vi "record.vi"(0 "Camera in":refnum<class "Camera.lvclass">, 5 "num_images":u32=1, 7 "record_mode":T1(ring), 9 "file_path":path, 11 "error in (no error)":errorcluster) -> (4 "Camera out":refnum<class "Camera.lvclass">, 15 "error out":errorcluster)   [LabVIEW 2020, in "Camera.lvclass"]
doc: "Creates, configures, and starts a new recorder instance. The entire camera configuration must be\nset before calling record.vi. The set_exposure_time.vi is the only exception. This function\nhas no effect on the recorder object and can be called during the recording."
uses:
  Camera.lvclass
  Camera.lvclass/Camera.ctl
  Recorder.lvlib
  GeneralCameraControl.lvlib
  RecordingControl.lvlib
  ImageSensor.lvlib
  Convert.lvlib
panel:
  out "filemode_no_overwrite":bool
  out "blocking_int":bool
  out "recType_int":u16
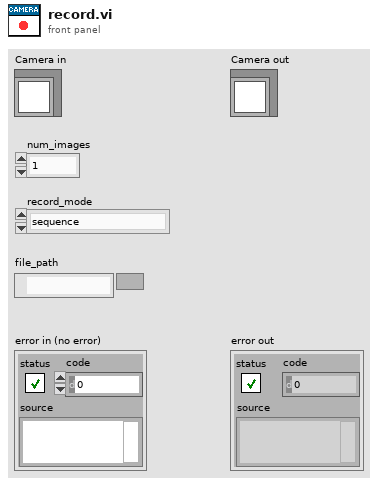
[diagram p1: front panel]
types:
  T1 = enum16{"sequence", "sequence non blocking", "ring buffer", "fifo", "sequence_dpcore", "sequence_non_blocking_dpcore", "ring_buffer_dpcore", "fifo_dpcore", "tif", "multitif", "pcoraw", "b16", "dicom", "multidicom"}
  T2 = map{enum16{"Undefined", "Mono8", "Mono16", "BGRA8", "RGBA8", "BGRA16", "RGBA16", "CompressedMono8"}, bool}
  T3 = cluster{"wSensorTypeDESC":u16, "wSensorSubTypeDESC":u16, "wMaxHorzResStdDESC":u16, "wMaxVertResStdDESC":u16, "wMaxHorzResExtDESC":u16, "wMaxVertResExtDESC":u16, "wDynResDESC":u16, "wMaxBinHorzDESC":u16, "wBinHorzSteppingDESC":u16, "wMaxBinVertDESC":u16, "wBinVertSteppingDESC":u16, "wRoiHorStepsDESC":u16, "wRoiVertStepsDESC":u16, "wNumADCsDESC":u16, "wMinSizeHorzDESC":u16, "dwPixelRateDESC":u32[], "wConvFactDESC":u16[], "sCoolingSetpoints":i16[], "wSoftRoiHorStepsDESC":u16, "wSoftRoiVertStepsDESC":u16, "wIRDESC":u16, "wMinSizeVertDESC":u16, "dwMinDelayDESC":u32, "dwMaxDelayDESC":u32, "dwMinDelayStepDESC":u32, "dwMinExposureDESC":u32, "dwMaxExposureDESC":u32, "dwMinExposureStepDESC":u32, "dwMinDelayIRDESC":u32, "dwMaxDelayIRDESC":u32, "dwMinExposureIRDESC":u32, "dwMaxExposureIRDESC":u32, "wTimeTableDESC":u16, "wDoubleImageDESC":u16, "sMinCoolSetDESC":i16, "sMaxCoolSetDESC":i16, "sDefaultCoolSetDESC":i16, "wPowerDownModeDESC":u16, "wOffsetRegulationDESC":u16, "wColorPatternDESC":u16, "wPatternTypeDESC":u16, "wNumCoolingSetpoints":u16, "dwGeneralCapsDESC1":u32, "dwGeneralCapsDESC2":u32, "dwExtSyncFrequency":u32[], "dwGeneralCapsDESC3":u32, "dwGeneralCapsDESC4":u32}
  T4 = cluster{"iConversionFactor":i32, "iDataBits":i32, "iSensorInfoBits":i32, "iDarkOffset":i32, "strColorCoeff":dbl[], "iCamNum":i32, "hCamera":u64}
  T5 = map{enum16{"Undefined", "Mono8", "Mono16", "BGRA8", "RGBA8", "BGRA16", "RGBA16", "CompressedMono8"}, u64}
  T6 = enum16{"Undefined", "Mono8", "Mono16", "BGRA8", "RGBA8", "BGRA16", "RGBA16", "CompressedMono8"}
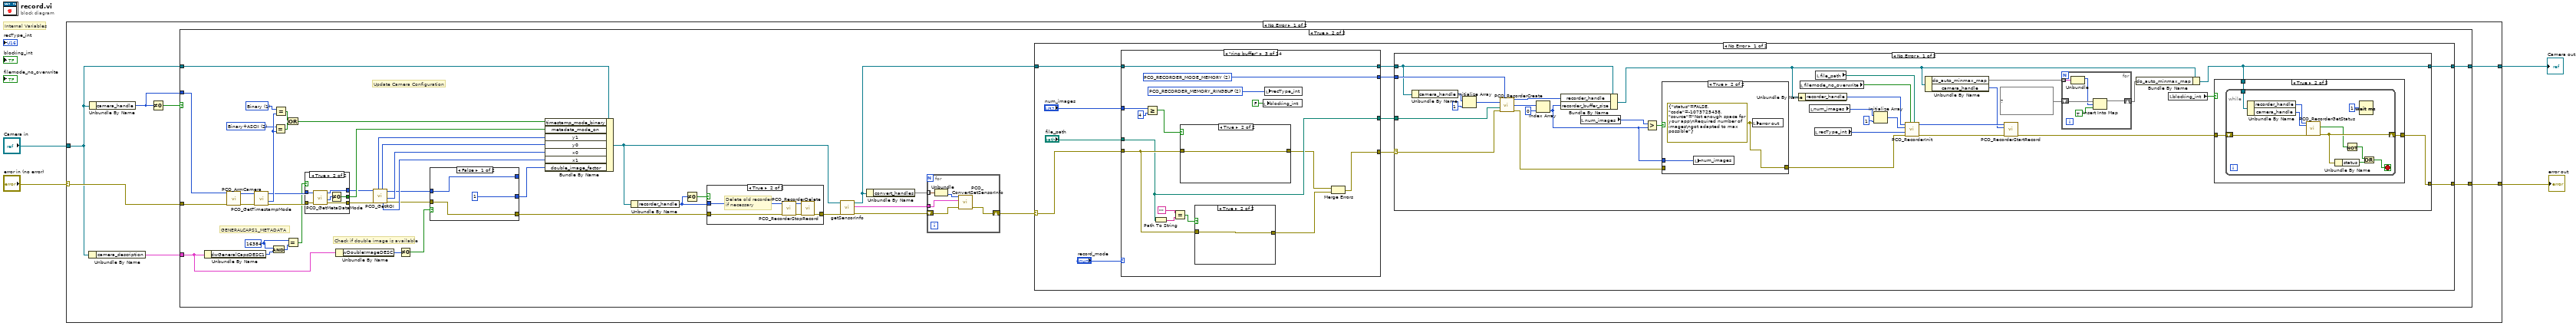
[diagram p0: block diagram]
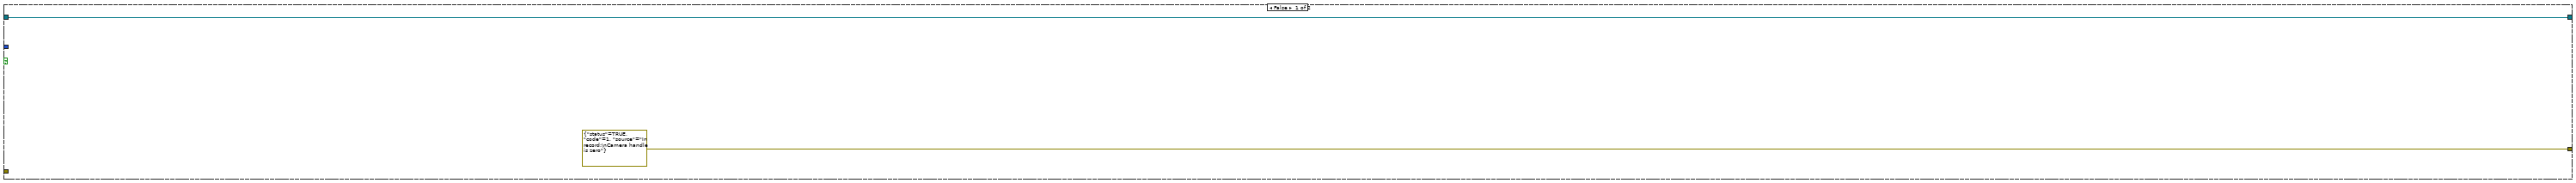
[diagram p2: hidden frame]
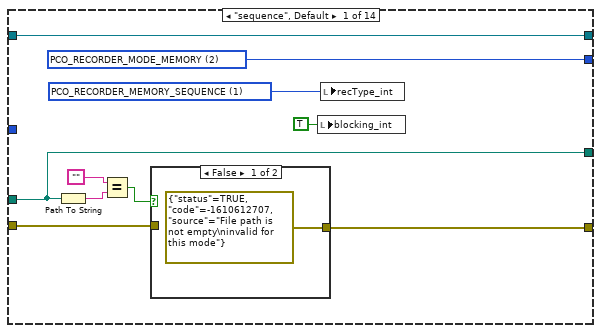
[diagram p6: hidden frame]
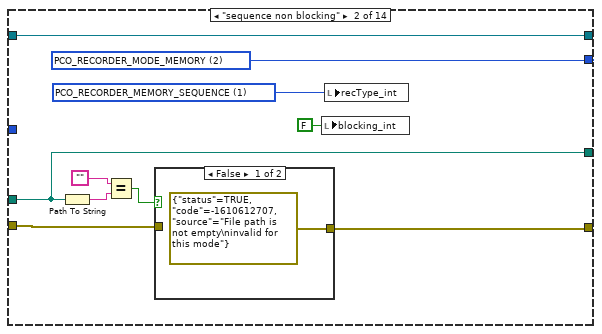
[diagram p8: hidden frame]
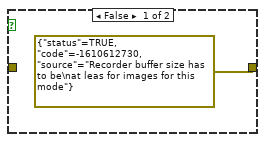
[diagram p10: hidden frame]
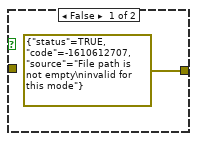
[diagram p11: hidden frame]
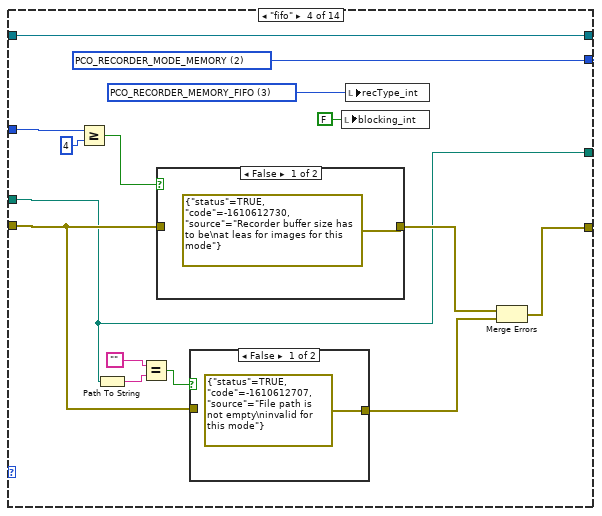
[diagram p12: hidden frame]
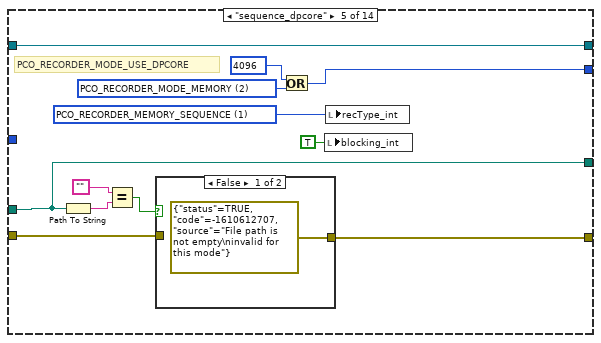
[diagram p15: hidden frame]
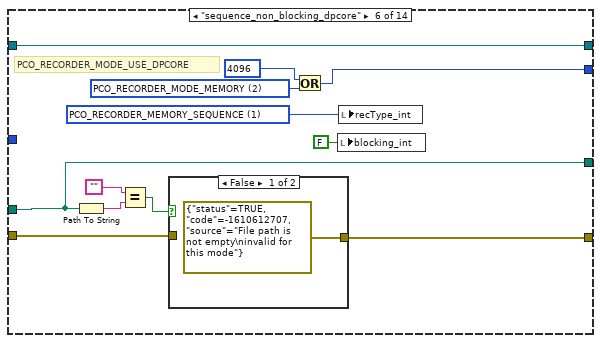
[diagram p17: hidden frame]
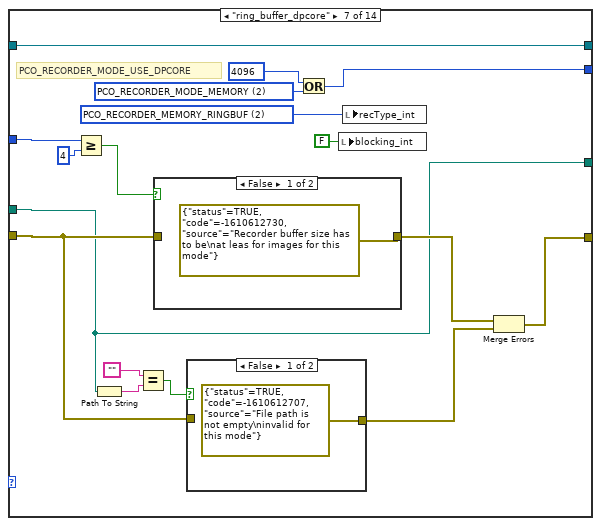
[diagram p19: hidden frame]
diagram:
  # "Internal Variables"
  n1 = case shown="No Error" "error in (no error)" {
    selector: "error in (no error)" -> [w7 w405]
    tunnel: [w10 w405] -> w3
    tunnel: [w9 w404] -> w1
    tunnel: "Camera in" -> [w6 w404]
    frame No Error {
      n2 = Unbundle By Name(w6) -> ("camera_description"=w5:T3)
      n3 = Unbundle By Name(w6) -> ("camera_handle"=w8:u64)
      n4 = Not Equal To 0?(x=w8) -> (x != 0?=w11:bool)
      n5 = case shown="True" w11 {
        tunnel: [errorcluster {"status"=TRUE, "code"=1, "source"="In record:\nCamera handle is zero"} ("error constant") w16] -> w10
        tunnel: w7 -> [_ w54]
        tunnel: w6 -> [w12 w51]
        tunnel: [w12 w14] -> w9
        tunnel: w8 -> [_ w55]
        tunnel: w5 -> [_ w31]
        frame False {
        }
        frame True {
          w40 = u32 16384 ("dwGeneralCapsDESC1")
          w48 = u16 2 items=["OFF", "Binary", "Binary+ASCII", "ASCII"] ("wTimeStampMode")
          w50 = u16 1 items=["OFF", "Binary", "Binary+ASCII", "ASCII"] ("wTimeStampMode")
          # "Update Camera Configuration"
          # "Check if double image is available"
          # "GENERALCAPS1_METADATA"
          n6 = Unbundle By Name(w31) -> ("dwGeneralCapsDESC1"=w42:u32)
          n7 = call "PCO_ArmCamera.vi"("error in (no error)"=w54, "ph"=w55) -> ("error out"=w53:errorcluster, "ph out"=w52:u64)  [unwired: 7 in, 1 out]
          n8 = call "PCO_GetTimestampMode.vi"("error in (no error)"=w53, "ph"=w52) -> ("error out"=w43:errorcluster, "wTimeStampMode"=w49:u16, "ph out"=w44:u64)  [unwired: 6 in, 1 out]
          n9 = And(x=w40, y=w42) -> (x .and. y?=w41:u32)
          n10 = Equal?(x=w48, y=w49) -> (x = y?=w47:bool)
          n11 = Equal?(x=w50, y=w49) -> (x = y?=w46:bool)
          n12 = Or(x=w46, y=w47) -> (x .or. y?=w45:bool)
          n13 = Equal?(x=w40, y=w41) -> (x = y?=w39:bool)
          n14 = case shown="True" w39 {
            tunnel: w44 -> [w395 w403]
            tunnel: w43 -> [w396 w402]
            tunnel: [w395 w401] -> w37
            tunnel: [w396 w400] -> w36
            tunnel: [FALSE w398] -> w38
            frame False {
            }
            frame True {
              n15 = call "PCO_GetMetaDataMode.vi"("error in (no error)"=w402, "ph"=w403) -> ("error out"=w400:errorcluster, "wMetaDataMode"=w399:u16, "ph out"=w401:u64)  [unwired: 4 in, 3 out]
              n16 = Not Equal To 0?(x=w399) -> (x != 0?=w398:bool)
            }
          }
          n17 = Unbundle By Name(w31) -> ("wDoubleImageDESC"=w30:u16)
          n18 = call "PCO_GetROI.vi"("error in (no error)"=w36, "ph"=w37) -> ("error out"=w28:errorcluster, "wRoiX0"=w33:u16, "ph out"=w27:u64, "wRoiX1"=w32:u16, "wRoiY0"=w35:u16, "wRoiY1"=w34:u16)  [unwired: 3 in, 1 out]
          n19 = Not Equal To 0?(x=w30) -> (x != 0?=w29:bool)
          n20 = case shown="False" w29 {
            tunnel: w28 -> [w383 w392]
            tunnel: w27 -> [w384 w391]
            tunnel: [u16 1 ("double_image_factor") w388] -> w26
            tunnel: [w383 w387] -> w25
            tunnel: [w384 w386] -> _
            frame False {
            }
            frame True {
              n21 = call "PCO_GetDoubleImageMode.vi"("error in (no error)"=w392, "ph"=w391) -> ("error out"=w387:errorcluster, "wDoubleImage"=w390:u16, "ph out"=w386:u64)  [unwired: 6 in, 1 out]
              n22 = Not Equal To 0?(x=w390) -> (x != 0?=w389:bool)
              n23 = case shown="True" w389 {
                tunnel: [u16 1 ("double_image_factor") u16 2 ("double_image_factor")] -> w388
                frame False {
                }
                frame True {
                }
              }
            }
          }
          n24 = Bundle By Name(cluster=w51, "timestamp_mode_binary"=w45, "metadata_mode_on"=w38, "y1"=w34, "y0"=w35, "x0"=w33, "x1"=w32, "double_image_factor"=w26) -> (w21:refnum<class "Camera.lvclass">)
          n25 = Unbundle By Name(w21) -> ("recorder_handle"=w23:u64)
          n26 = Not Equal To 0?(x=w23) -> (x != 0?=w24:bool)
          n27 = case shown="True" w24 {
            tunnel: w23 -> [_ w381]
            tunnel: w25 -> [w377 w382]
            tunnel: [w377 w378] -> w22
            frame False {
            }
            frame True {
              # "Delete old recorder\nif necessary"
              n28 = call "PCO_RecorderStopRecord.vi"("error in (no error)"=w382, "phRec"=w381) -> ("error out"=w380:errorcluster, "phRec out"=w379:u64)  [unwired: 7 in, 1 out]
              n29 = call "PCO_RecorderDelete.vi"("error in (no error)"=w380, "phRec"=w379) -> ("error out"=w378:errorcluster)  [unwired: 8 in, 1 out]
            }
          }
          n30 = call-dynamic "getSensorInfo.vi"("error in (no error)"=w22, "Camera in"=w21) -> ("error out"=w18:errorcluster, "PCO_SensorInfo"=w19:T4, "Camera out"=w15:refnum<class "Camera.lvclass">)  [unwired: 7 in]
          n31 = Unbundle By Name(w15) -> ("convert_handles"=w20:T5)
          n32 = for {
            tunnel: w20 -> [w376] mode=indexing
            tunnel: w19 -> [w374]
            shift-right: [w372] -> w17
            shift-left: w18 -> [w373]
            n33 = Unbundle(w376) -> (w375:u64)  [unwired: 1 out]
            n34 = call "PCO_ConvertSetSensorInfo.vi"("error in (no error)"=w373, "strSensorInfo"=w374, "ph"=w375) -> ("error out"=w372:errorcluster)  [unwired: 6 in, 2 out]
          }
          n35 = case shown="No Error" w17 {
            selector: w17 -> [w59 w371]
            tunnel: [w56 w371] -> w16
            tunnel: w15 -> [w65 w370]
            tunnel: [w57 w370] -> w14
            frame No Error {
              n36 = case shown="\"ring buffer\"" "record_mode" {
                tunnel: w65 -> [w128 w145 w155 w167 w188 w201 w217 w235 w260 w277 w295 w314 w333 w354]
                tunnel: "file_path" -> [w127 w137 w151 w170 w191 w203 w216 w236 w259 w281 w299 w319 w338 w357]
                tunnel: "num_images" -> [_ _ w162 w172 _ _ w220 w241 _ _ _ _ _ _]
                tunnel: [w124 w138 w148 w169 w190 w200 w215 w237 w258 w278 w298 w316 w335 w352] -> w60
                tunnel: [w129 w136 w154 w168 w186 w202 w214 w238 w262 w276 w296 w315 w334 w355] -> w62
                tunnel: [w128 w145 w155 w167 w188 w201 w217 w235 w260 w277 w295 w314 w333 w354] -> w61
                tunnel: [w127 w137 w151 w170 w191 w203 w216 w236 w257 w279 w297 w317 w336 w353] -> w58
                tunnel: w59 -> [w125 w139 w152 w171 w192 w204 w221 w240 w263 w280 w300 w318 w337 w356]
                frame "sequence", Default {
                  w129 = u16 2 items=["PCO_RECORDER_MODE_FILE"=1, "PCO_RECORDER_MODE_MEMORY"=2, "PCO_RECORDER_MODE_CAMRAM"=3] ("wRecMode")
                  w130 = u16 1 items=["PCO_RECORDER_MEMORY_SEQUENCE"=1, "PCO_RECORDER_MEMORY_RINGBUF"=2, "PCO_RECORDER_MEMORY_FIFO"=3] ("wRecType")
                  n37 = Path To String(path=w127) -> (string=w132:string)
                  n38 = Equal?(x="", y=w132) -> (x = y?=w126:bool)
                  n39 = case shown="False" w126 {
                    tunnel: w125 -> [_ w135]
                    tunnel: [errorcluster {"status"=TRUE, "code"=-1610612707, "source"="File path is not empty\ninvalid for this mode"} ("error constant") w135] -> w124
                    frame False {
                    }
                    frame True {
                    }
                  }
                  n40 = local write "blocking_int"(TRUE ("blocking_int")) -> ()
                  n41 = local write "recType_int"(w130) -> ()
                }
                frame "sequence non blocking" {
                  w136 = u16 2 items=["PCO_RECORDER_MODE_FILE"=1, "PCO_RECORDER_MODE_MEMORY"=2, "PCO_RECORDER_MODE_CAMRAM"=3] ("wRecMode")
                  w141 = u16 1 items=["PCO_RECORDER_MEMORY_SEQUENCE"=1, "PCO_RECORDER_MEMORY_RINGBUF"=2, "PCO_RECORDER_MEMORY_FIFO"=3] ("wRecType")
                  n42 = Path To String(path=w137) -> (string=w143:string)
                  n43 = Equal?(x="", y=w143) -> (x = y?=w140:bool)
                  n44 = case shown="False" w140 {
                    tunnel: w139 -> [_ w147]
                    tunnel: [errorcluster {"status"=TRUE, "code"=-1610612707, "source"="File path is not empty\ninvalid for this mode"} ("error constant") w147] -> w138
                    frame False {
                    }
                    frame True {
                    }
                  }
                  n45 = local write "blocking_int"(FALSE ("blocking_int")) -> ()
                  n46 = local write "recType_int"(w141) -> ()
                }
                frame "ring buffer" {
                  w154 = u16 2 items=["PCO_RECORDER_MODE_FILE"=1, "PCO_RECORDER_MODE_MEMORY"=2, "PCO_RECORDER_MODE_CAMRAM"=3] ("wRecMode")
                  w157 = u16 2 items=["PCO_RECORDER_MEMORY_SEQUENCE"=1, "PCO_RECORDER_MEMORY_RINGBUF"=2, "PCO_RECORDER_MEMORY_FIFO"=3] ("wRecType")
                  n47 = Greater Or Equal?(x=w162, y=u32 4) -> (x >= y?=w153:bool)
                  n48 = Path To String(path=w151) -> (string=w159:string)
                  n49 = Equal?(x="", y=w159) -> (x = y?=w156:bool)
                  n50 = case shown="True" w153 {
                    tunnel: w152 -> [_ w164]
                    tunnel: [errorcluster {"status"=TRUE, "code"=-1610612730, "source"="Recorder buffer size has to be\nat leas for images for this mode"} ("error constant") w164] -> w150
                    frame False {
                    }
                    frame True {
                    }
                  }
                  n51 = case shown="True" w156 {
                    tunnel: w152 -> [_ w166]
                    tunnel: [errorcluster {"status"=TRUE, "code"=-1610612707, "source"="File path is not empty\ninvalid for this mode"} ("error constant") w166] -> w149
                    frame False {
                    }
                    frame True {
                    }
                  }
                  n52 = local write "blocking_int"(FALSE ("blocking_int")) -> ()
                  n53 = local write "recType_int"(w157) -> ()
                  n54 = Merge Errors(w150, w149) -> (w148:errorcluster)
                }
                frame "fifo" {
                  w168 = u16 2 items=["PCO_RECORDER_MODE_FILE"=1, "PCO_RECORDER_MODE_MEMORY"=2, "PCO_RECORDER_MODE_CAMRAM"=3] ("wRecMode")
                  w177 = u16 3 items=["PCO_RECORDER_MEMORY_SEQUENCE"=1, "PCO_RECORDER_MEMORY_RINGBUF"=2, "PCO_RECORDER_MEMORY_FIFO"=3] ("wRecType")
                  n55 = Greater Or Equal?(x=w172, y=u32 4) -> (x >= y?=w175:bool)
                  n56 = Path To String(path=w170) -> (string=w179:string)
                  n57 = Equal?(x="", y=w179) -> (x = y?=w176:bool)
                  n58 = case shown="False" w175 {
                    tunnel: w171 -> [_ w183]
                    tunnel: [errorcluster {"status"=TRUE, "code"=-1610612730, "source"="Recorder buffer size has to be\nat leas for images for this mode"} ("error constant") w183] -> w174
                    frame False {
                    }
                    frame True {
                    }
                  }
                  n59 = case shown="False" w176 {
                    tunnel: w171 -> [_ w185]
                    tunnel: [errorcluster {"status"=TRUE, "code"=-1610612707, "source"="File path is not empty\ninvalid for this mode"} ("error constant") w185] -> w173
                    frame False {
                    }
                    frame True {
                    }
                  }
                  n60 = local write "blocking_int"(FALSE ("blocking_int")) -> ()
                  n61 = local write "recType_int"(w177) -> ()
                  n62 = Merge Errors(w174, w173) -> (w169:errorcluster)
                }
                frame "sequence_dpcore" {
                  w187 = u16 2 items=["PCO_RECORDER_MODE_FILE"=1, "PCO_RECORDER_MODE_MEMORY"=2, "PCO_RECORDER_MODE_CAMRAM"=3] ("wRecMode")
                  w194 = u16 1 items=["PCO_RECORDER_MEMORY_SEQUENCE"=1, "PCO_RECORDER_MEMORY_RINGBUF"=2, "PCO_RECORDER_MEMORY_FIFO"=3] ("wRecType")
                  # "PCO_RECORDER_MODE_USE_DPCORE"
                  n63 = Path To String(path=w191) -> (string=w196:string)
                  n64 = Equal?(x="", y=w196) -> (x = y?=w193:bool)
                  n65 = case shown="False" w193 {
                    tunnel: w192 -> [_ w199]
                    tunnel: [errorcluster {"status"=TRUE, "code"=-1610612707, "source"="File path is not empty\ninvalid for this mode"} ("error constant") w199] -> w190
                    frame False {
                    }
                    frame True {
                    }
                  }
                  n66 = Or(x=u16 4096 ("dimension size"), y=w187) -> (x .or. y?=w186:u16)
                  n67 = local write "blocking_int"(TRUE ("blocking_int")) -> ()
                  n68 = local write "recType_int"(w194) -> ()
                }
                frame "sequence_non_blocking_dpcore" {
                  w205 = u16 2 items=["PCO_RECORDER_MODE_FILE"=1, "PCO_RECORDER_MODE_MEMORY"=2, "PCO_RECORDER_MODE_CAMRAM"=3] ("wRecMode")
                  w208 = u16 1 items=["PCO_RECORDER_MEMORY_SEQUENCE"=1, "PCO_RECORDER_MEMORY_RINGBUF"=2, "PCO_RECORDER_MEMORY_FIFO"=3] ("wRecType")
                  # "PCO_RECORDER_MODE_USE_DPCORE"
                  n69 = Path To String(path=w203) -> (string=w210:string)
                  n70 = Equal?(x="", y=w210) -> (x = y?=w207:bool)
                  n71 = case shown="False" w207 {
                    tunnel: w204 -> [_ w213]
                    tunnel: [errorcluster {"status"=TRUE, "code"=-1610612707, "source"="File path is not empty\ninvalid for this mode"} ("error constant") w213] -> w200
                    frame False {
                    }
                    frame True {
                    }
                  }
                  n72 = Or(x=u16 4096 ("dimension size"), y=w205) -> (x .or. y?=w202:u16)
                  n73 = local write "blocking_int"(FALSE ("blocking_int")) -> ()
                  n74 = local write "recType_int"(w208) -> ()
                }
                frame "ring_buffer_dpcore" {
                  w218 = u16 2 items=["PCO_RECORDER_MODE_FILE"=1, "PCO_RECORDER_MODE_MEMORY"=2, "PCO_RECORDER_MODE_CAMRAM"=3] ("wRecMode")
                  w226 = u16 2 items=["PCO_RECORDER_MEMORY_SEQUENCE"=1, "PCO_RECORDER_MEMORY_RINGBUF"=2, "PCO_RECORDER_MEMORY_FIFO"=3] ("wRecType")
                  # "PCO_RECORDER_MODE_USE_DPCORE"
                  n75 = Greater Or Equal?(x=w220, y=u32 4) -> (x >= y?=w224:bool)
                  n76 = Path To String(path=w216) -> (string=w228:string)
                  n77 = Equal?(x="", y=w228) -> (x = y?=w225:bool)
                  n78 = case shown="False" w224 {
                    tunnel: w221 -> [_ w232]
                    tunnel: [errorcluster {"status"=TRUE, "code"=-1610612730, "source"="Recorder buffer size has to be\nat leas for images for this mode"} ("error constant") w232] -> w223
                    frame False {
                    }
                    frame True {
                    }
                  }
                  n79 = case shown="False" w225 {
                    tunnel: w221 -> [_ w234]
                    tunnel: [errorcluster {"status"=TRUE, "code"=-1610612707, "source"="File path is not empty\ninvalid for this mode"} ("error constant") w234] -> w222
                    frame False {
                    }
                    frame True {
                    }
                  }
                  n80 = Or(x=u16 4096 ("dimension size"), y=w218) -> (x .or. y?=w214:u16)
                  n81 = local write "blocking_int"(FALSE ("blocking_int")) -> ()
                  n82 = local write "recType_int"(w226) -> ()
                  n83 = Merge Errors(w223, w222) -> (w215:errorcluster)
                }
                frame "fifo_dpcore" {
                  w242 = u16 2 items=["PCO_RECORDER_MODE_FILE"=1, "PCO_RECORDER_MODE_MEMORY"=2, "PCO_RECORDER_MODE_CAMRAM"=3] ("wRecMode")
                  w247 = u16 3 items=["PCO_RECORDER_MEMORY_SEQUENCE"=1, "PCO_RECORDER_MEMORY_RINGBUF"=2, "PCO_RECORDER_MEMORY_FIFO"=3] ("wRecType")
                  # "PCO_RECORDER_MODE_USE_DPCORE"
                  n84 = Greater Or Equal?(x=w241, y=u32 4) -> (x >= y?=w245:bool)
                  n85 = Path To String(path=w236) -> (string=w249:string)
                  n86 = Equal?(x="", y=w249) -> (x = y?=w246:bool)
                  n87 = case shown="False" w245 {
                    tunnel: w240 -> [_ w253]
                    tunnel: [errorcluster {"status"=TRUE, "code"=-1610612730, "source"="Recorder buffer size has to be\nat leas for images for this mode"} ("error constant") w253] -> w244
                    frame False {
                    }
                    frame True {
                    }
                  }
                  n88 = case shown="False" w246 {
                    tunnel: w240 -> [_ w255]
                    tunnel: [errorcluster {"status"=TRUE, "code"=-1610612707, "source"="File path is not empty\ninvalid for this mode"} ("error constant") w255] -> w243
                    frame False {
                    }
                    frame True {
                    }
                  }
                  n89 = Or(x=u16 4096 ("dimension size"), y=w242) -> (x .or. y?=w238:u16)
                  n90 = local write "blocking_int"(FALSE ("blocking_int")) -> ()
                  n91 = local write "recType_int"(w247) -> ()
                  n92 = Merge Errors(w244, w243) -> (w237:errorcluster)
                }
                frame "tif" {
                  w261 = u16 1 items=["PCO_RECORDER_FILE_TIF"=1, "PCO_RECORDER_FILE_MULTITIF"=2, "PCO_RECORDER_FILE_PCORAW"=3, "PCO_RECORDER_FILE_B16"=4, "PCO_RECORDER_FILE_DICOM"=5, "PCO_RECORDER_FILE_MULTIDICOM"=6] ("wRecType")
                  w262 = u16 1 items=["PCO_RECORDER_MODE_FILE"=1, "PCO_RECORDER_MODE_MEMORY"=2, "PCO_RECORDER_MODE_CAMRAM"=3] ("wRecMode")
                  # "Get parent of file path if possible"
                  n93 = Path To String(path=w259) -> (string=w266:string)
                  n94 = Not Equal?(x="", y=w266) -> (x != y?=w264:bool)
                  n95 = case shown="False" w264 {
                    tunnel: w263 -> [_ w272]
                    tunnel: [errorcluster {"status"=TRUE, "code"=-1610612707, "source"="File path is empty\nspecify valid path for\nrecord to file"} ("error constant") w272] -> w258
                    frame False {
                    }
                    frame True {
                    }
                  }
                  n96 = local write "filemode_no_overwrite"(TRUE ("blocking_int")) -> ()
                  n97 = local write "blocking_int"(FALSE ("blocking_int")) -> ()
                  n98 = local write "recType_int"(w261) -> ()
                  n99 = Strip Path(path=w259) -> (stripped path=w268:path)  [unwired: 1 out]
                  n100 = Equal?(x=path "", y=w268) -> (x = y?=w269:bool)
                  n101 = case shown="False" w269 {
                    tunnel: w268 -> [w273 _]
                    tunnel: w259 -> [_ w274]
                    tunnel: [w273 w274] -> w257
                    frame False {
                    }
                    frame True {
                    }
                  }
                }
                frame "multitif" {
                  w282 = u16 2 items=["PCO_RECORDER_FILE_TIF"=1, "PCO_RECORDER_FILE_MULTITIF"=2, "PCO_RECORDER_FILE_PCORAW"=3, "PCO_RECORDER_FILE_B16"=4, "PCO_RECORDER_FILE_DICOM"=5, "PCO_RECORDER_FILE_MULTIDICOM"=6] ("wRecType")
                  w276 = u16 1 items=["PCO_RECORDER_MODE_FILE"=1, "PCO_RECORDER_MODE_MEMORY"=2, "PCO_RECORDER_MODE_CAMRAM"=3] ("wRecMode")
                  # "Get parent of file path if possible"
                  n102 = Path To String(path=w281) -> (string=w285:string)
                  n103 = Not Equal?(x="", y=w285) -> (x != y?=w283:bool)
                  n104 = case shown="False" w283 {
                    tunnel: w280 -> [_ w291]
                    tunnel: [errorcluster {"status"=TRUE, "code"=-1610612707, "source"="File path is empty\nspecify valid path for\nrecord to file"} ("error constant") w291] -> w278
                    frame False {
                    }
                    frame True {
                    }
                  }
                  n105 = local write "filemode_no_overwrite"(TRUE ("blocking_int")) -> ()
                  n106 = local write "blocking_int"(FALSE ("blocking_int")) -> ()
                  n107 = local write "recType_int"(w282) -> ()
                  n108 = Strip Path(path=w281) -> (stripped path=w287:path)  [unwired: 1 out]
                  n109 = Equal?(x=path "", y=w287) -> (x = y?=w288:bool)
                  n110 = case shown="False" w288 {
                    tunnel: w287 -> [w292 _]
                    tunnel: w281 -> [_ w293]
                    tunnel: [w292 w293] -> w279
                    frame False {
                    }
                    frame True {
                    }
                  }
                }
                frame "pcoraw" {
                  w301 = u16 3 items=["PCO_RECORDER_FILE_TIF"=1, "PCO_RECORDER_FILE_MULTITIF"=2, "PCO_RECORDER_FILE_PCORAW"=3, "PCO_RECORDER_FILE_B16"=4, "PCO_RECORDER_FILE_DICOM"=5, "PCO_RECORDER_FILE_MULTIDICOM"=6] ("wRecType")
                  w296 = u16 1 items=["PCO_RECORDER_MODE_FILE"=1, "PCO_RECORDER_MODE_MEMORY"=2, "PCO_RECORDER_MODE_CAMRAM"=3] ("wRecMode")
                  # "Get parent of file path if possible"
                  n111 = Path To String(path=w299) -> (string=w304:string)
                  n112 = Not Equal?(x="", y=w304) -> (x != y?=w302:bool)
                  n113 = case shown="False" w302 {
                    tunnel: w300 -> [_ w310]
                    tunnel: [errorcluster {"status"=TRUE, "code"=-1610612707, "source"="File path is empty\nspecify valid path for\nrecord to file"} ("error constant") w310] -> w298
                    frame False {
                    }
                    frame True {
                    }
                  }
                  n114 = local write "filemode_no_overwrite"(TRUE ("blocking_int")) -> ()
                  n115 = local write "blocking_int"(FALSE ("blocking_int")) -> ()
                  n116 = local write "recType_int"(w301) -> ()
                  n117 = Strip Path(path=w299) -> (stripped path=w306:path)  [unwired: 1 out]
                  n118 = Equal?(x=path "", y=w306) -> (x = y?=w307:bool)
                  n119 = case shown="True" w307 {
                    tunnel: w306 -> [w311 _]
                    tunnel: w299 -> [_ w312]
                    tunnel: [w311 w312] -> w297
                    frame False {
                    }
                    frame True {
                    }
                  }
                }
                frame "b16" {
                  w320 = u16 4 items=["PCO_RECORDER_FILE_TIF"=1, "PCO_RECORDER_FILE_MULTITIF"=2, "PCO_RECORDER_FILE_PCORAW"=3, "PCO_RECORDER_FILE_B16"=4, "PCO_RECORDER_FILE_DICOM"=5, "PCO_RECORDER_FILE_MULTIDICOM"=6] ("wRecType")
                  w315 = u16 1 items=["PCO_RECORDER_MODE_FILE"=1, "PCO_RECORDER_MODE_MEMORY"=2, "PCO_RECORDER_MODE_CAMRAM"=3] ("wRecMode")
                  # "Get parent of file path if possible"
                  n120 = Path To String(path=w319) -> (string=w323:string)
                  n121 = Not Equal?(x="", y=w323) -> (x != y?=w321:bool)
                  n122 = case shown="False" w321 {
                    tunnel: w318 -> [_ w329]
                    tunnel: [errorcluster {"status"=TRUE, "code"=-1610612707, "source"="File path is empty\nspecify valid path for\nrecord to file"} ("error constant") w329] -> w316
                    frame False {
                    }
                    frame True {
                    }
                  }
                  n123 = local write "filemode_no_overwrite"(TRUE ("blocking_int")) -> ()
                  n124 = local write "blocking_int"(FALSE ("blocking_int")) -> ()
                  n125 = local write "recType_int"(w320) -> ()
                  n126 = Strip Path(path=w319) -> (stripped path=w325:path)  [unwired: 1 out]
                  n127 = Equal?(x=path "", y=w325) -> (x = y?=w326:bool)
                  n128 = case shown="True" w326 {
                    tunnel: w325 -> [w330 _]
                    tunnel: w319 -> [_ w331]
                    tunnel: [w330 w331] -> w317
                    frame False {
                    }
                    frame True {
                    }
                  }
                }
                frame "dicom" {
                  w339 = u16 5 items=["PCO_RECORDER_FILE_TIF"=1, "PCO_RECORDER_FILE_MULTITIF"=2, "PCO_RECORDER_FILE_PCORAW"=3, "PCO_RECORDER_FILE_B16"=4, "PCO_RECORDER_FILE_DICOM"=5, "PCO_RECORDER_FILE_MULTIDICOM"=6] ("wRecType")
                  w334 = u16 1 items=["PCO_RECORDER_MODE_FILE"=1, "PCO_RECORDER_MODE_MEMORY"=2, "PCO_RECORDER_MODE_CAMRAM"=3] ("wRecMode")
                  # "Get parent of file path if possible"
                  n129 = Path To String(path=w338) -> (string=w342:string)
                  n130 = Not Equal?(x="", y=w342) -> (x != y?=w340:bool)
                  n131 = case shown="False" w340 {
                    tunnel: w337 -> [_ w348]
                    tunnel: [errorcluster {"status"=TRUE, "code"=-1610612707, "source"="File path is empty\nspecify valid path for\nrecord to file"} ("error constant") w348] -> w335
                    frame False {
                    }
                    frame True {
                    }
                  }
                  n132 = local write "filemode_no_overwrite"(TRUE ("blocking_int")) -> ()
                  n133 = local write "blocking_int"(FALSE ("blocking_int")) -> ()
                  n134 = local write "recType_int"(w339) -> ()
                  n135 = Strip Path(path=w338) -> (stripped path=w344:path)  [unwired: 1 out]
                  n136 = Equal?(x=path "", y=w344) -> (x = y?=w345:bool)
                  n137 = case shown="True" w345 {
                    tunnel: w344 -> [w349 _]
                    tunnel: w338 -> [_ w350]
                    tunnel: [w349 w350] -> w336
                    frame False {
                    }
                    frame True {
                    }
                  }
                }
                frame "multidicom" {
                  w358 = u16 6 items=["PCO_RECORDER_FILE_TIF"=1, "PCO_RECORDER_FILE_MULTITIF"=2, "PCO_RECORDER_FILE_PCORAW"=3, "PCO_RECORDER_FILE_B16"=4, "PCO_RECORDER_FILE_DICOM"=5, "PCO_RECORDER_FILE_MULTIDICOM"=6] ("wRecType")
                  w355 = u16 1 items=["PCO_RECORDER_MODE_FILE"=1, "PCO_RECORDER_MODE_MEMORY"=2, "PCO_RECORDER_MODE_CAMRAM"=3] ("wRecMode")
                  # "Get parent of file path if possible"
                  n138 = Path To String(path=w357) -> (string=w361:string)
                  n139 = Not Equal?(x="", y=w361) -> (x != y?=w359:bool)
                  n140 = case shown="False" w359 {
                    tunnel: w356 -> [_ w367]
                    tunnel: [errorcluster {"status"=TRUE, "code"=-1610612707, "source"="File path is empty\nspecify valid path for\nrecord to file"} ("error constant") w367] -> w352
                    frame False {
                    }
                    frame True {
                    }
                  }
                  n141 = local write "filemode_no_overwrite"(TRUE ("blocking_int")) -> ()
                  n142 = local write "blocking_int"(FALSE ("blocking_int")) -> ()
                  n143 = local write "recType_int"(w358) -> ()
                  n144 = Strip Path(path=w357) -> (stripped path=w363:path)  [unwired: 1 out]
                  n145 = Equal?(x=path "", y=w363) -> (x = y?=w364:bool)
                  n146 = case shown="True" w364 {
                    tunnel: w363 -> [w368 _]
                    tunnel: w357 -> [_ w369]
                    tunnel: [w368 w369] -> w353
                    frame False {
                    }
                    frame True {
                    }
                  }
                }
              }
              n147 = case shown="No Error" w60 {
                selector: w60 -> [w92 w122]
                tunnel: [w73 w122] -> w56
                tunnel: w61 -> [w72 w123]
                tunnel: [w67 w123] -> w57
                tunnel: w62 -> [w93 _]
                tunnel: w58 -> [w91 _]
                frame No Error {
                  n148 = Unbundle By Name(w72) -> ("camera_handle"=w98:u64)
                  n149 = Initialize Array(w98, 1 ("dimension size")) -> (w97:u64[])
                  n150 = call "PCO_RecorderCreate.vi"("wRecMode"=w93, "phCamArr"=w97, "szDrive"=w91, "error in (no error)"=w92) -> ("phRec out"=w94:u64, "dwMaxImgCountArr"=w95:u32[], "error out"=w85:errorcluster)  [unwired: 8 in, 1 out]
                  n151 = Index Array(array=w95, index=0) -> (element=w88:u32)
                  n152 = Bundle By Name(cluster=w72, "recorder_handle"=w94, "recorder_buffer_size"=w88) -> (w69:refnum<class "Camera.lvclass">)
                  n153 = local read "num_images"() -> (w90:u32)
                  n154 = Greater?(x=w90, y=w88) -> (0:w89:bool)
                  n155 = case shown="True" w89 {
                    tunnel: w88 -> [_ w121]
                    tunnel: w85 -> [w119 _]
                    tunnel: [w119 w120] -> w84
                    frame False {
                    }
                    frame True {
                      w120 = errorcluster {"status"=FALSE, "code"=-1073725438, "source"="Not enough space for your app\nRequired number of images\ngot adapted to max possible"} ("error constant")
                      n156 = local write "num_images"(w121) -> ()
                      n157 = local write "error out"(w120) -> ()
                    }
                  }
                  n158 = Unbundle By Name(w69) -> ("recorder_handle"=w87:u64)
                  n159 = local read "filemode_no_overwrite"() -> (w79:bool)
                  n160 = local read "num_images"() -> (w83:u32)
                  n161 = local read "recType_int"() -> (w81:u16)
                  n162 = local read "file_path"() -> (w80:path)
                  n163 = Initialize Array(w83, 1 ("dimension size")) -> (w82:u32[])
                  n164 = call "PCO_RecorderInit.vi"("szFilePath"=w80, "noOverwrite"=w79, "error in (no error)"=w84, "wType"=w81, "dwImgCountArr"=w82, "phRec"=w87) -> ("error out"=w78:errorcluster, "phRec out"=w77:u64)  [unwired: 3 in, 1 out]
                  n165 = Unbundle By Name(w69) -> ("do_auto_minmax_map"=w71:T2, "camera_handle"=w76:u64)
                  n166 = call "PCO_RecorderStartRecord.vi"("error in (no error)"=w78, "phCam"=w76, "phRec"=w77) -> ("error out"=w74:errorcluster)  [unwired: 6 in, 2 out]
                  n167 = for {
                    tunnel: w71 -> [w104] mode=indexing
                    shift-right: [w100] -> w68
                    shift-left: T2 {} ("do_auto_minmax_map") -> [w103]
                    n168 = Unbundle(w104) -> (w102:T6)  [unwired: 1 out]
                    n169 = Insert Into Map(map in=w103, key=w102, value=TRUE ("status")) -> (map out=w100:T2)  [unwired: 2 out]
                  }
                  n170 = Bundle By Name(cluster=w69, "do_auto_minmax_map"=w68) -> (w67:refnum<class "Camera.lvclass">)
                  n171 = local read "blocking_int"() -> (w75:bool)
                  n172 = case shown="True" w75 {
                    tunnel: w74 -> [w105 w108]
                    tunnel: w67 -> [_ w107]
                    tunnel: [w105 w106] -> w73
                    frame False {
                    }
                    frame True {
                      n173 = while {
                        shift-right: [w112] -> w106
                        shift-left: w108 -> [w115]
                        tunnel: w107 -> [w118]
                        stop <- w113 stop-if-true
                        n174 = Unbundle By Name(w118) -> ("recorder_handle"=w117:u64, "camera_handle"=w116:u64)
                        n175 = call "PCO_RecorderGetStatus.vi"("phRec"=w117, "phCam"=w116, "error in (no error)"=w115) -> ("bIsRunning"=w110:bool, "error out"=w112:errorcluster)  [unwired: 5 in, 10 out]
                        n176 = Unbundle By Name(w112) -> ("status"=w114:bool)
                        n177 = Not(x=w110) -> (.not. x?=w109:bool)
                        n178 = Wait (ms)(milliseconds to wait=u32 1) -> ()  [unwired: 1 out]
                        n179 = Or(x=w109, y=w114) -> (x .or. y?=w113:bool)
                      }
                    }
                  }
                }
                frame Error {
                }
              }
            }
            frame Error {
            }
          }
        }
      }
    }
    frame Error {
    }
  }
  "error out" <- w3
  "Camera out" <- w1
